vi "WriteTree.vi"(8 "error in":errorcluster, 11 "repository in":refnum<class "modification container.lvclass">) -> (0 "error out":errorcluster, 2 "root":T1, 3 "repository out":refnum<class "NISE_CEF_Repository.lvclass">)   [LabVIEW 2013, in "modification container.lvclass"]
doc: "Transfers information between the repo and the tree control. This method should be called after the custom views are called or saving to disk."
uses:
  modification container.lvclass
  <vilib>/NI/Configuration Framework/Repository/NISE_CEF_Repository.lvclass
  <vilib>/NI/Configuration Framework/Node/NodeRef.ctl
  <vilib>/NI/Configuration Framework/Node/NISE_CEF_Node.lvclass
  collection/VI modification collection.lvclass
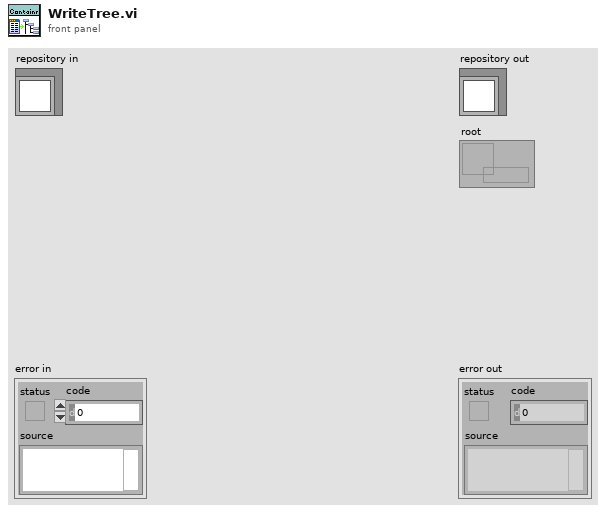
[diagram p1: front panel]
types:
  T1 = typedef "NISE_CEF_Node.lvclass/NodeRef.ctl" = refnum<data-value>
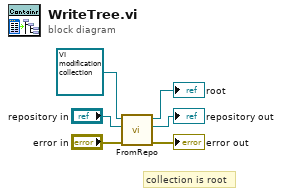
[diagram p0: block diagram]
diagram:
  # "collection is root"
  n1 = call-dynamic "FromRepo.vi"("error in"="error in", "repository in"="repository in", "node in"=refnum<class "VI modification collection.lvclass"> refnum ("VI modification collection.lvclass")) -> ("error out"=→"error out":errorcluster, "repository out"=→"repository out":refnum<class "NISE_CEF_Repository.lvclass">, "node"=→"root":T1)  [unwired: 6 in]
